vi "AutoBike FPGA.vi"() -> ()   [LabVIEW 2016]
doc: "The roboRIO FPGA Shipping Personality. This personality supports:\n- 8 Analog Input channels with 1 sample\n- 2 Analog Output channels with 1 sample\n- 30 Digital I/O channels with 1 sample\n- 1 RSL channel\n- 4 Relay channels\n- 1 Button\n- 3 LEDs\n- 1 Accelerometer\n- 13 PWM channels\n- 6 Encoder channels\n- 2 SPI channels\n- 2 I2C channels\n- 2 UART channels\n- 1 CAN channel\n- 2 Analog Input Interrupt\n- 5 Digital Input Interrupt\n- 1 Timer Interrupt"
uses:
  Sub VIs for FPGA/SubVIs needed for the customize FPGA VI/Utilities/Start Boolean.ctl
  <vilib>/Platform/TimedLoop/XDataNode/timing_clust.ctl
  <vilib>/Platform/TimedLoop/XDataNode/nitl_modes.ctl
  <vilib>/Platform/TimedLoop/XDataNode/wakeup.ctl
  <vilib>/rvi/Analysis/control/PID/Typedef/niFpgaPID_PIGains.ctl
  <vilib>/rvi/Analysis/control/PID/Typedef/niFpgaPID_OutputRange.ctl
  <vilib>/rvi/Emulation/niFpgaGetClockAttributes.vi
  <vilib>/rvi/Emulation/niFpgaSctlEmulationGetInTimedLoop.vi
  <vilib>/rvi/Emulation/niFpgaEmulationReportErrorSimple.vi
  <vilib>/rvi/eio/common/nirviEmuTemplateMethod_errors.vi
  <vilib>/rvi/Emulation/niFpgaCriticalErrorInLSC.vi
  <vilib>/rvi/Emulation/niFpgaProcessEmulError.vi
  <vilib>/rvi/Emulation/niFpgaEmulationIsFPGAContextNoSignature.vi
  <vilib>/rvi/errors/niFpgaSetErrorForExecOnDevCompSimple.vi
  <vilib>/rvi/eio/common/nirviEmuReportErrorAndStop.vi
  <vilib>/rvi/DataTransferAndStorage/Container/Common/niFpgaContainerGetUniqueNameForEmu.vi
  <vilib>/rvi/FIFO/Fifo_Resource/nirvififoEmulationSetSize.vi
  <vilib>/rvi/FIFO/Fifo_Resource/nirviFifoEmulationQueueMgr.vi
  <instcachedir>/0/nirviFifoEmulationQueueMgr_E5CAEC123FF24DC58D834DCA3CDAA9B5.lvgen/nirviFifoEmulationQueueMgr_E5CAEC123FF24DC58D834DCA3CDAA9B5_002.vi
  <vilib>/Utility/error.llb/Clear Errors.vi
  <vilib>/rvi/FIFO/Fifo_Resource/nirvififoEmulationCreateLock.vi
  <vilib>/rvi/FIFO/Fifo_Resource/nirvififoEmulationObtainLock.vi
  <vilib>/rvi/FIFO/Fifo_Resource/nirvififoEmulationReleaseLock.vi
  <vilib>/rvi/occurrence/nirviWaitOnOccurrenceBase.vi
  <vilib>/rvi/errors/nirviReportUnexpectedCaseInternalError.vi
  <vilib>/rvi/errors/nirviReportUnexpectedCaseInternalError (U32).vi
  <vilib>/rvi/FIFO/Fifo_Resource/nirvififoEmulationDetermineInputValidOut.vi
  <vilib>/rvi/Analysis/control/PID/SubVIs/niFpgaPID_PIWrapper.vi
  <vilib>/rvi/DataTransferAndStorage/Container/Common/niFpgaContainerSetEmuInfo.vi
  <vilib>/eio/EIONode/EIONode.xnode
  <vilib>/rvi/DataTransferAndStorage/Container/XNode/niFpgaContainer.xnode
  <vilib>/rvi/FIFO/Fifo_Resource/nirvififoEmulationRead.vi
  <vilib>/rvi/FIFO/Fifo_Resource/nirvififoEmulationWrite.vi
  <vilib>/Platform/TimedLoop/XDataNode/XDataNode.xnode
  <vilib>/rvi/LocalResourceManager/LocalResourceManager.xnode
  <vilib>/Platform/TimedLoop/XDataNode/XDNodeRunTimeDep.lvlib
panel:
  out "error":sgl
  in  "Control Loop Duty Cycle":sgl
  in  "Control Loop Direction":bool
  in  "Front Panel Duty Cycle":sgl
  in  "Front Panel Direction":bool
  in  "Shut Down BW":bool
  out "Duty cycle (steering)":sgl
  out "Steering angle(deg)":sgl
  in  "Duty Cycle in":sgl
  out "Current speed":sgl
  out "Duty cycle (BW)":sgl
  in  "Reference speed in km/h":sgl=15.0
  out "Filtered data":i32
  out "Value Channel 0":i32
  out "Channel 4 position":i32
  out "Channel 5 position":i32
  out "Channel 6 position":i32
  out "Channel 7 position":i32
  out "Position":i64
  in  "Stop encoder":bool
  in  "Reset counter":bool
  in  "Stop direction switch":bool
  in  "Switch direction":bool
  out "HallSensorValue":u8
  in  "Stop Hallsensor":bool
  out "dt":u32
  out "DIO.SPI_CS3:0.IN":u8 format="%08b"
  in  "DIO.SPI_CS3:0.DIR":u8 format="%08b"
  in  "DIO.SPI_CS3:0.OUT":u8 format="%08b"
  in  "IRQ.TIMER.SETTIME":T1
  in  "IRQ.TIMER.WRITE":u32
  out "IRQ.TIMER.READ":u32
  in  "IRQ.DI_BTN.NO":u8
  in  "IRQ.DI_BTN.CNT":u32
  in  "IRQ.DI_BTN.FALL":bool
  in  "IRQ.DI_BTN.RISE":bool
  in  "IRQ.DI_BTN.ENA":bool
  in  "IRQ.AI_B_0.HYSTERESIS":u16=17
  in  "IRQ.AI_B_1.HYSTERESIS":u16=17
  in  "IRQ.AI_B_1.NO":u8
  in  "IRQ.AI_B_0.NO":u8
  in  "IRQ.AI_B_1.THRESHOLD":u16
  in  "IRQ.AI_B_0.THRESHOLD":u16
  in  "IRQ.AI_B_3:0.CNFG":u8 format="%.0b"
  in  "IRQ.DIO_B_0.NO":u8
  in  "IRQ.DIO_B_1.NO":u8
  in  "IRQ.DIO_B_2.NO":u8
  in  "IRQ.DIO_B_3.NO":u8
  in  "IRQ.DIO_B_3.CNT":u32
  in  "IRQ.DIO_B_2.CNT":u32
  in  "IRQ.DIO_B_1.CNT":u32
  in  "IRQ.DIO_B_0.CNT":u32
  in  "IRQ.DIO_B_7:0.FALL":u8 format="%08b"
  in  "IRQ.DIO_B_7:0.RISE":u8 format="%08b"
  in  "IRQ.DIO_B_7:0.ENA":u8 format="%08b"
  in  "SPI.SPI.IRQ.NO":u8=15
  in  "SPI.B.IRQ.NO":u8=15
  out "DIO.DIO_9:8.IN":u8 format="%08b"
  in  "ENC.DIO_3.CNFG":u8 format="%08b"
  out "ENC.DIO_3.CNTR":u32
  out "ENC.DIO_3.STAT":u8 format="%08b"
  in  "ENC.DIO_4.CNFG":u8 format="%08b"
  out "ENC.DIO_4.CNTR":u32
  out "ENC.DIO_4.STAT":u8 format="%08b"
  in  "DIO.DIO_9:8.OUT":u8 format="%08b"
  in  "DIO.DIO_9:8.DIR":u8 format="%08b"
  in  "ENC.DIO_2.CNFG":u8 format="%08b"
  out "ENC.DIO_2.CNTR":u32
  out "ENC.DIO_2.STAT":u8 format="%08b"
  out "ENC.DIO_1.STAT":u8 format="%08b"
  out "ENC.DIO_1.CNTR":u32
  in  "ENC.DIO_1.CNFG":u8 format="%08b"
  out "DIO.DIO_7:0.IN":u8 format="%08b"
  in  "SYS.SELECTDIO":u8 format="%08b"
  in  "DIO.DIO_7:0.DIR":u8 format="%08b"
  in  "DIO.DIO_7:0.OUT":u8 format="%08b"
  out "ENC.DIO_0.STAT":u8 format="%08b"
  out "ENC.DIO_0.CNTR":u32
  in  "ENC.DIO_0.CNFG":u8 format="%08b"
  out "DI.BTN":u8 format="%08b"
  in  "DO.LED 5:0":u8 format="%06b"
  in  "DO.RSL.OUT":bool
  out "SPI.SPI.STAT":u8 format="%08b"
  in  "SPI.SPI.GO":T1
  in  "SPI.SPI.CNT":u16
  in  "SPI.SPI.CNFG":u16 format="%016b"
  out "SPI.SPI.DATI":u16
  in  "SPI.SPI.DATO":u16
  out "I2C.I2C.DATI":u8
  out "I2C.I2C.STAT":u8 format="%08b"
  in  "I2C.I2C.DATO":u8
  in  "I2C.I2CADDR":u8 format="%08b"
  in  "I2C.I2C.CNTR":u8
  in  "I2C.I2C.CNTL":u8 format="%08b"
  in  "I2C.I2C.CNFG":u8 format="%08b"
  in  "I2C.I2C.GO":T1
  out "ACC.Z.VAL":u16
  out "ACC.Y.VAL":u16
  out "ACC.X.VAL":u16
  in  "DO.RELAY.OUT":u8 format="%08b"
  out "SYS.ACC.RDY":bool
  out "SYS.RDY":bool
  in  "PWM.PWM_5.MAX":u16
  in  "PWM.PWM_5.CMP":u16
  in  "PWM.PWM_5.CNFG":u8 format="%08b"
  in  "PWM.PWM_5.CS":u8
  out "PWM.PWM_5.CNTR":u16
  in  "PWM.PWM_6.MAX":u16
  in  "PWM.PWM_6.CMP":u16
  in  "PWM.PWM_6.CNFG":u8 format="%08b"
  in  "PWM.PWM_6.CS":u8
  out "PWM.PWM_6.CNTR":u16
  in  "PWM.PWM_7.MAX":u16
  in  "PWM.PWM_7.CMP":u16
  in  "PWM.PWM_7.CNFG":u8 format="%08b"
  in  "PWM.PWM_7.CS":u8
  out "PWM.PWM_7.CNTR":u16
  in  "PWM.PWM_8.MAX":u16
  in  "PWM.PWM_8.CMP":u16
  in  "PWM.PWM_8.CNFG":u8 format="%08b"
  in  "PWM.PWM_8.CS":u8
  out "PWM.PWM_8.CNTR":u16
  in  "PWM.PWM_9.MAX":u16
  in  "PWM.PWM_9.CMP":u16
  in  "PWM.PWM_9.CNFG":u8 format="%08b"
  in  "PWM.PWM_9.CS":u8
  out "PWM.PWM_9.CNTR":u16
  in  "PWM.PWM_4.MAX":u16
  in  "PWM.PWM_4.CMP":u16
  in  "PWM.PWM_4.CNFG":u8 format="%08b"
  in  "PWM.PWM_4.CS":u8
  out "PWM.PWM_4.CNTR":u16
  in  "PWM.PWM_3.MAX":u16
  in  "PWM.PWM_3.CMP":u16
  in  "PWM.PWM_3.CNFG":u8 format="%08b"
  in  "PWM.PWM_3.CS":u8
  out "PWM.PWM_3.CNTR":u16
  in  "PWM.PWM_2.MAX":u16
  in  "PWM.PWM_2.CMP":u16
  in  "PWM.PWM_2.CNFG":u8 format="%08b"
  in  "PWM.PWM_2.CS":u8
  out "PWM.PWM_2.CNTR":u16
  in  "PWM.PWM_1.MAX":u16
  in  "PWM.PWM_1.CMP":u16
  in  "PWM.PWM_1.CNFG":u8 format="%08b"
  in  "PWM.PWM_1.CS":u8
  out "PWM.PWM_1.CNTR":u16
  out "PWM.PWM_0.CNTR":u16
  in  "PWM.PWM_0.CS":u8
  in  "PWM.PWM_0.CNFG":u8 format="%08b"
  in  "PWM.PWM_0.CMP":u16
  in  "PWM.PWM_0.MAX":u16
  in  "AO.B_0.VAL":u16
  in  "AO.B_1.VAL":u16
  in  "AO.SYS.GO":T1
  out "AO.SYS.STAT":bool
  out "AI.B_0.VAL":u16
  out "AI.B_1.VAL":u16
  out "AI.B_2.VAL":u16
  out "AI.B_3.VAL":u16
  out "AI.AI_0.VAL":u16
  out "AI.AI_1.VAL":u16
  out "AI.AI_2.VAL":u16
  out "AI.AI_3.VAL":u16
  out "SYS.AI.RDY":bool
  in  "SYS.SELECTB":u8 format="%08b"
  in  "DIO.B_7:0.OUT":u8 format="%08b"
  in  "DIO.B_7:0.DIR":u8 format="%08b"
  out "DIO.B_7:0.IN":u8 format="%08b"
  in  "DIO.B_15:8.OUT":u8 format="%08b"
  in  "DIO.B_15:8.DIR":u8 format="%08b"
  out "DIO.B_15:8.IN":u8 format="%08b"
  in  "SPI.B.DATO":u16
  out "SPI.B.DATI":u16
  in  "SPI.B.CNFG":u16 format="%016b"
  in  "SPI.B.CNT":u16
  in  "SPI.B.GO":T1
  out "SPI.B.STAT":u8 format="%08b"
  in  "PWM.B_0.MAX":u16
  in  "PWM.B_0.CMP":u16
  in  "PWM.B_0.CNFG":u8 format="%08b"
  in  "PWM.B_0.CS":u8
  out "PWM.B_0.CNTR":u16
  in  "PWM.B_1.CMP":u16
  in  "PWM.B_1.MAX":u16
  out "PWM.B_1.CNTR":u16
  in  "PWM.B_1.CNFG":u8 format="%08b"
  in  "PWM.B_1.CS":u8
  in  "PWM.B_2.CMP":u16
  in  "PWM.B_2.MAX":u16
  out "PWM.B_2.CNTR":u16
  in  "PWM.B_2.CNFG":u8 format="%08b"
  in  "PWM.B_2.CS":u8
  in  "I2C.B.DATO":u8
  out "I2C.B.DATI":u8
  in  "I2C.B.ADDR":u8 format="%08b"
  in  "I2C.B.CNTR":u8
  in  "I2C.B.CNTL":u8 format="%08b"
  out "I2C.B.STAT":u8 format="%08b"
  in  "I2C.B.CNFG":u8 format="%08b"
  in  "I2C.B.GO":T1
  in  "ENC.B.CNFG":u8 format="%08b"
  out "ENC.B.CNTR":u32
  out "ENC.B.STAT":u8 format="%08b"
  # "System"
  # "Onboard Devices"
  # "Connector B"
  # "DIO"
  # "SPI"
  # "PWM"
  # "I2C"
  # "AI"
  # "RELAY"
  # "RSL"
  # "Accelerometer"
  # "SPI Master"
  # "Analog Input"
  # "Analog Output"
  # "Digital I/O"
  # "Counters / PWM"
  # "Digital I/O"
  # "Encoders"
  # "IO Configuration"
  # "Buttons & LEDs"
  # "SPI CS DIO"
  # "Analog Interrupt"
  # "Digital Interrupt"
  # "Encoders"
  # "IO Configuration"
  # "Button Interrupt"
  # "I2C Master"
  # "FPGA Timer"
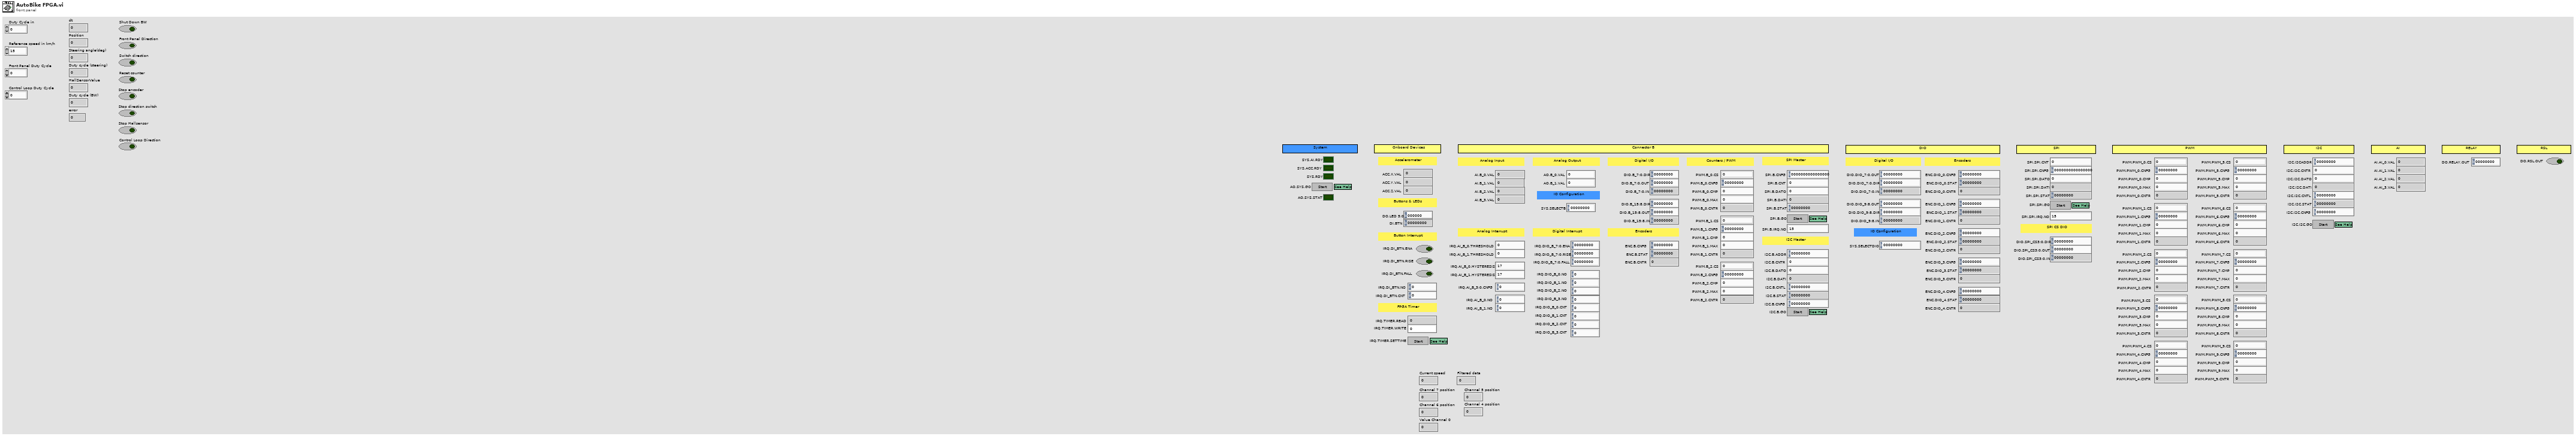
[diagram p1: front panel]
types:
  T1 = typedef "Start Boolean.ctl" = bool
  T2 = typedef "XDNodeRunTimeDep.lvlib/timing_clust.ctl" = cluster{"Expected End [f-1]":u64, "Actual End [f-1]":u64, "Finished Late? [f-1]":bool, "Expected End [i-1]":u64, "Actual End [i-1]":u64, "Finished Late? [i-1]":bool, "Expected Start [i]":u64, "Actual Start [i]":u64, "Expected Start [f]":u64, "Actual Start [f]":u64, "Source Name":string, "Structure Name":string, "Period":i64, "Deadline":i64, "Offset":i64, "Start":i64, "Priority":i32, "Timeout":i32, "Mode":T3, "Wakeup Reason":T4, "Error":errorcluster, "Source Type":string, "Secondary Source Type":string, "Global End Time":u64, "Global Start Time":u64, "Frame Duration":u64, "Iteration Duration":u64, "Assigned CPU":i32, "I/O Scan Engine Mode":u32}
  T3 = typedef "XDNodeRunTimeDep.lvlib/nitl_modes.ctl" = enum32{"No Change", "Process missed periods, maintain original phase", "Discard missed periods, maintain original phase", "Process missed periods, ignore original phase", "Discard missed periods, ignore original phase"}
  T4 = typedef "XDNodeRunTimeDep.lvlib/wakeup.ctl" = enum32{"Normal", "Aborted", "Asynchronous wakeup", "Timing source error", "Timed loop error", "Timeout"}
  T5 = typedef "niFpgaPID_OutputRange.ctl" = cluster{"output high (Inf)":sgl, "output low (-Inf)":sgl}
  T6 = typedef "niFpgaPID_PIGains.ctl" = cluster{"proportional gain":sgl, "integral gain":sgl}
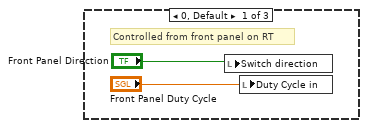
[diagram p2: hidden frame]
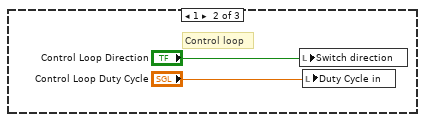
[diagram p3: hidden frame]
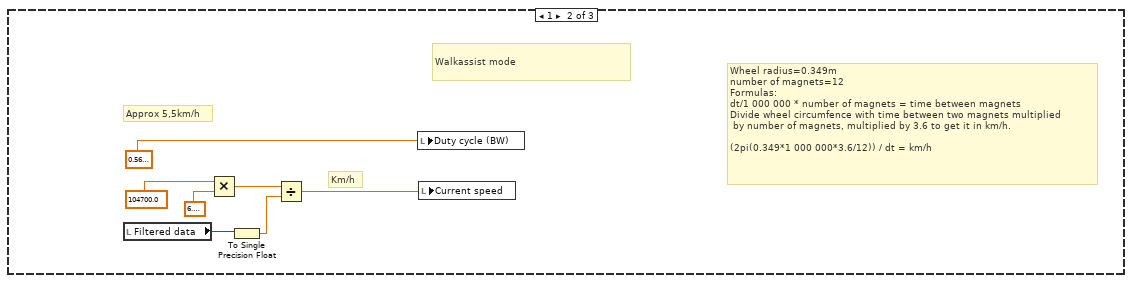
[diagram p4: hidden frame]
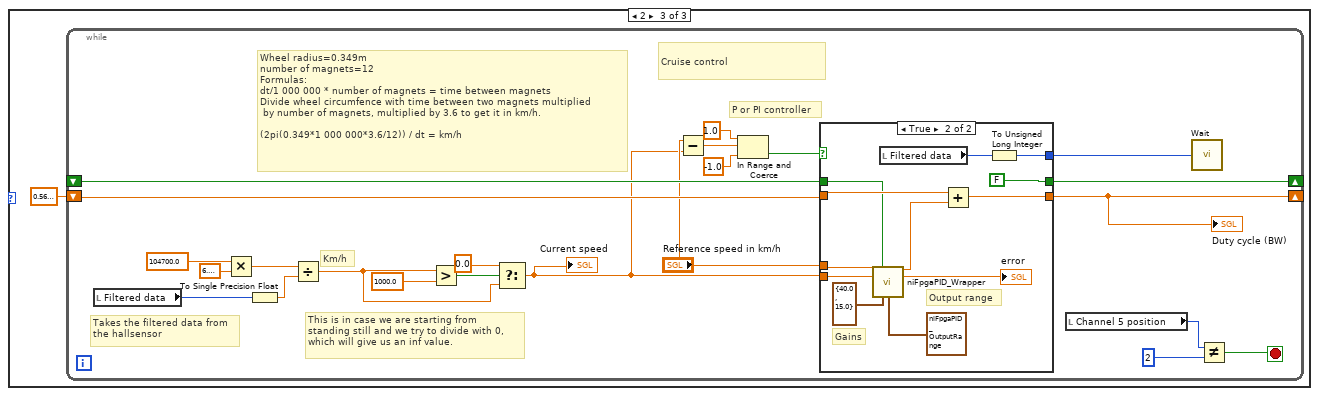
[diagram p5: hidden frame]
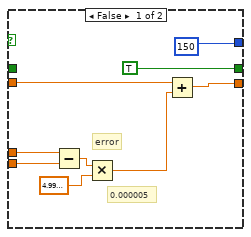
[diagram p6: hidden frame]
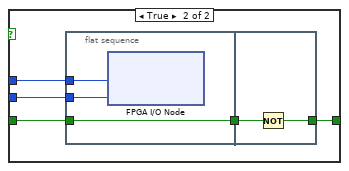
[diagram p13: hidden frame]
diagram:
  # "DONT USE PWN 1, IT IS CONNECTED ON THREE OUTS"
  # "The accelerometer nodes take some time before the FPGA can first read the values. This is because it takes time to read from the accelerometer. An iteration of the While Loop will not complete until the accelerometer values have been read.\n\nAfter the completion of the first iteration of the While Loop, all indicators have valid values."
  # "The analog output nodes take some time before the FPGA write the values to the pins. The GO and STAT registers are used to handshake between the FPGA and host. When the host wants the values to be written, the host sets the GO register to TRUE. If the host reads the STAT register before setting the value of the GO register, it can wait for the value of the STAT register to invert. The value inversion tells the host that the output values have been written."
  # "The FPGA timer fires the interrupt request (IRQ) when TIMER.Read counts down to zero. If TIMER.Read is not zero, it counts down to one per microsecond."
  # "The analog input nodes take some time before the FPGA can first read the values. This is because it takes time to set up the Analog-to-Digital converter (ADC) and convert the first reading. An iteration of the While Loop will not complete until all the analog input channels have been sampled.\n\nAfter the completion of the first iteration of the While Loop, all indicators have valid values."
  # "Note: On some hardware a \"ghosting effect\" may occur on any unconnected AI channels. For example, if channel AI0 is connected and channels AI1~AI7 are not connected the the value read at AI0 may be seen on indicators AI1~AI7. This is common for hardware that use a multiplexed (MUXed) Analog-to-Digital converter (ADC), because the input analog signal is used to charge a capacitor which does not discharge before the unconnected channel is read.\n\nYou can hide the \"ghosting effect\" by using an mask register. This register is used to decide when the indicator should be updated."
  # "The only interface that sends interrupts to the RT side. Timer interrupts, analog input interrupts, digital input interrupts, and SPI interrupt share this interface.\n\nAll interrupts work in sequence. One interrupt waits until the previous interrupt request (IRQ) gets acknowledged on the RT side."
  # "NOTE: The SYS.RDY boolean MUST exist and must become TRUE at some point otherwise the myRIO API will not function correctly."
  # "There is some delay between when the FPGA code starts and the analog inputs, accelerometer, and scaling values outputs are valid. If the host wants to ensure that there are valid values in theses registers it should wait for each subsystem to finish its initialization process. \n\nWhen all subsystems have finished initializinig, the SYS.RDY indicator will be true, which can be polled by the host to determine the status of the FPGA. Alternatively, the host can poll the individual SYS.xx.RDY indicators to determine the status of the individual subsystems.\n\nThis loop continues indefinitely, essentially making SYS.RDY a read-only register."
  n1 = flat-sequence {
    tunnel: [i64 0] -> w2
    tunnel: [TRUE ("DIO/DIO3")] -> w1
    tunnel: w2 -> [w29]
    tunnel: w1 -> [w28]
    frame #0 {
      # "Initialise"
    }
    frame #1 {
      n2 = while {
        shift-right: [w49] -> _
        shift-left: w28 -> [w51]
        stop <- "Stop Hallsensor" stop-if-true
        n3 = flat-sequence {
          tunnel: w51 -> [w54]
          tunnel: [w54] -> w48
          tunnel: [u8 0] -> w47
          tunnel: [w52] -> w46
          tunnel: w48 -> [w59]
          tunnel: w47 -> [w57]
          tunnel: w46 -> [w56]
          tunnel: [w58] -> w45
          tunnel: [w55] -> w44
          tunnel: [w81] -> w49
          tunnel: w45 -> [w81]
          tunnel: [w80] -> w43
          tunnel: w44 -> [w78]
          frame #0 {
            n4 = call "Tick Count4"() -> ("Tick Count(uSec)"=w52:u32)
          }
          frame #1 {
            n5 = node-c288() -> (w61:T2)  [unwired: 1 in]
            n6 = timed-loop {
              shift-right: [w65] -> _
              shift-left: w57 -> [w62]
              shift-right: [w70] -> w58
              shift-left: w59 -> [w73]
              timing: w61 -> [_]
              timing-out: [_] -> w60
              tunnel: w56 -> [w72]
              tunnel: [w72] -> w55
              stop <- w64 stop-if-true
              # "Calculates the time it takes to collect 2 rises, i.e one magnet"
              # "Reads the output from the hallsensor and outputs the number of change in rises"
              # "Hallsensor counter"
              n7 = xnode "FPGA I/O Node"() -> ("DIO/DIO8"=w70:bool)  [unwired: 1 in, 1 out]
              n8 = Exclusive Or(1:w73, 2:w70) -> (0:w68:bool)
              n9 = Not And(1:TRUE ("y"), 2:w70) -> (0:w69:bool)
              n10 = And(x=w69, y=w68) -> (x .and. y?=w67:bool)
              n11 = Increment(x=w62) -> (x+1=w66:u8)
              n12 = Select(t=w66, s=w67, f=w62) -> (s? t:f=w65:u8)
              "HallSensorValue" <- w65
              n13 = Equal?(x=u8 2, y=w65) -> (x = y?=w64:bool)
            }
            n14 = node-c288(w60) -> ()
          }
          frame #2 {
            n15 = call "Tick Count"() -> ("Tick Count(uSec)"=w79:u32)
            n16 = Subtract(x=w79, y=w78) -> (x-y=w80:u32)
          }
        }
        n17 = To Long Integer(number=w43) -> (32bit integer=w42:i32)
        n18 = call "Median filter.vi"("Rawdata"=w42) -> ("Filtered element"=w39:i32)  [unwired: 10 in]
        n19 = Equal To 0?(x=w39) -> (x = 0?=w41:bool)
        n20 = Select(t=1, s=w41, f=w39) -> (s? t:f=→"Filtered data":i32)
      }
      n21 = node-c288() -> (w31:T2)  [unwired: 1 in]
      n22 = node-c288() -> (w27:T2)  [unwired: 1 in]
      n23 = timed-loop {
        shift-right: [w92] -> _
        shift-left: w29 -> [w83]
        shift-right: [w89] -> _
        shift-left: _ -> [w87]
        shift-right: [w88] -> _
        shift-left: _ -> [w86]
        timing: w31 -> [_]
        timing-out: [_] -> w30
        stop <- "Stop encoder" stop-if-true
        # "Decoder, reads both signals and check if there is any change to any of the channels, if there is a change current A channel\nis compared to previous B channel to determine which direction the motor is going and updates the position counter\naccordingly. The counter is resetted each time the Main VI is deployed."
        # "Motor Decoder"
        n24 = xnode "FPGA I/O Node"() -> ("DIO/DIO0"=w89:bool, "DIO/DIO1"=w88:bool)  [unwired: 2 in, 2 out]
        n25 = Exclusive Or(1:w86, 2:w89) -> (0:w85:bool)
        n26 = Select(t=i64 0, s="Reset counter", f=w83) -> (s? t:f=w91:i64)
        n27 = Exclusive Or(1:w87, 2:w89) -> (0:w99:bool)
        n28 = Exclusive Or(1:w86, 2:w88) -> (0:w98:bool)
        n29 = Or(x=w99, y=w98) -> (x .or. y?=w84:bool)
        n30 = Select(t=i64 1, s=w85, f=i64 -1) -> (s? t:f=w94:i64)
        n31 = Add(x=w94, y=w91) -> (x+y=w93:i64)
        n32 = Select(t=w93, s=w84, f=w91) -> (s? t:f=w92:i64)
        "Position" <- w92
      }
      n33 = timed-loop {
        timing: w27 -> [_]
        timing-out: [_] -> w26
        stop <- "Stop direction switch" stop-if-true
        # "Switch the direction of the steering\nmotor."
        # "Switch direction"
        n34 = xnode "FPGA I/O Node"("DIO/DIO2"="Switch direction") -> ()  [unwired: 1 in, 1 out]
      }
      n35 = node-c288(w26) -> ()
      n36 = node-c288(w30) -> ()
    }
  }
  n37 = while {
    stop <- FALSE stop-if-true
    # "PWM signal to steering motor"
    n38 = flat-sequence {
      tunnel: [w107] -> w104
      tunnel: [w112] -> w106
      tunnel: w104 -> [w109]
      tunnel: w106 -> [w114]
      frame #0 {
        w107 = u32 40000 ("Freq")
        # "40000 ticks=1kHz"
        n39 = call "Loop Timer3"("Count(Ticks)"=w107) -> ()  [unwired: 1 out]
      }
      frame #1 {
        # "Too make sure 0 duty \ncycle is generated"
        n40 = local read "Duty cycle (steering)"() -> (w110:sgl)
        n41 = To Single Precision Float(number=w109) -> (single precision float=w108:sgl)
        n42 = Not Equal To 0?(x=w110) -> (x != 0?=w111:bool)
        n43 = Multiply(x=w110, y=w108) -> (x*y=w113:sgl)
        n44 = xnode "FPGA I/O Node"("PWM/PWM0"=w111) -> ()  [unwired: 1 in, 1 out]
        n45 = To Unsigned Long Integer(number=w113) -> (unsigned 32bit integer=w112:u32)
      }
      frame #2 {
        n46 = call "Wait3"("Count(Ticks)"=w114) -> ()  [unwired: 1 out]
      }
      frame #3 {
        n47 = xnode "FPGA I/O Node"("PWM/PWM0"=FALSE ("PWM/PWM8")) -> ()  [unwired: 1 in, 1 out]
      }
    }
  }
  n48 = while {
    stop <- FALSE stop-if-true
    # "PWM signal to backwheel motor"
    n49 = flat-sequence {
      tunnel: [w121] -> w117
      tunnel: w117 -> [w124]
      frame #0 {
        # "80 000ticks=500Hz"
        n50 = call "Loop Timer2"("Count(Ticks)"=u32 80000) -> ()  [unwired: 1 out]
      }
      frame #1 {
        n51 = local read "Duty cycle (BW)"() -> (w119:sgl)
        n52 = xnode "FPGA I/O Node"("PWM/PWM8"=TRUE) -> ()  [unwired: 1 in, 1 out]
        n53 = Multiply(x=w119, y=sgl 80000.0) -> (x*y=w122:sgl)
        n54 = To Unsigned Long Integer(number=w122) -> (unsigned 32bit integer=w121:u32)
      }
      frame #2 {
        n55 = call "Wait2"("Count(Ticks)"=w124) -> ()  [unwired: 1 out]
      }
      frame #3 {
        n56 = xnode "FPGA I/O Node"("PWM/PWM8"=FALSE) -> ()  [unwired: 1 in, 1 out]
      }
    }
  }
  n57 = while {
    stop <- FALSE stop-if-true
    # "Backwheel motor control"
    n58 = local read "Channel 5 position"() -> (w126:i32)
    n59 = case shown="0, Default" w126 {
      frame 0, Default {
        # "Wheel radius=0.349m\nnumber of magnets=12\nFormulas:\ndt/1 000 000 * number of magnets = time between magnets\nDivide wheel circumfence with time between two magnets multiplied\n by number of magnets, multiplied by 3.6 to get it in km/h.\n\n(2pi(0.349*1 000 000*3.6/12)) / dt = km/h"
        # "Takes the filtered data from\nthe hallsensor"
        # "Km/h"
        # "Standing still"
        n60 = local read "Filtered data"() -> (w129:i32)
        n61 = Multiply(x=sgl 104700.0, y=sgl 6.2831855) -> (x*y=w135:sgl)
        n62 = To Single Precision Float(number=w129) -> (single precision float=w130:sgl)
        n63 = Divide(x=w135, y=w130) -> (x/y=w131:sgl)
        n64 = Greater?(x=w131, y=sgl 1000.0) -> (0:w133:bool)
        n65 = local write "Duty cycle (BW)"(sgl 0.5 ("Duty cycle out 2")) -> ()
        n66 = Select(t=sgl 0.0, s=w133, f=w131) -> (s? t:f=w128:sgl)
        n67 = local write "Current speed"(w128) -> ()
      }
      frame 1 {
        # "Wheel radius=0.349m\nnumber of magnets=12\nFormulas:\ndt/1 000 000 * number of magnets = time between magnets\nDivide wheel circumfence with time between two magnets multiplied\n by number of magnets, multiplied by 3.6 to get it in km/h.\n\n(2pi(0.349*1 000 000*3.6/12)) / dt = km/h"
        # "Walkassist mode"
        # "Approx 5,5km/h"
        # "Km/h"
        n68 = local read "Filtered data"() -> (w142:i32)
        n69 = Multiply(x=sgl 104700.0, y=sgl 6.2831855) -> (x*y=w143:sgl)
        n70 = To Single Precision Float(number=w142) -> (single precision float=w141:sgl)
        n71 = Divide(x=w143, y=w141) -> (x/y=w140:sgl)
        n72 = local write "Duty cycle (BW)"(sgl 0.56 ("Duty cycle out")) -> ()
        n73 = local write "Current speed"(w140) -> ()
      }
      frame 2 {
        n74 = while {
          shift-right: [w157] -> _
          shift-left: sgl 0.56 -> [w156]
          shift-right: [w155] -> _
          shift-left: _ -> [w154]
          stop <- w158 stop-if-true
          # "P or PI controller"
          # "This is in case we are starting from\nstanding still and we try to divide with 0, \nwhich will give us an inf value."
          # "Cruise control"
          # "Takes the filtered data from\nthe hallsensor"
          # "Wheel radius=0.349m\nnumber of magnets=12\nFormulas:\ndt/1 000 000 * number of magnets = time between magnets\nDivide wheel circumfence with time between two magnets multiplied\n by number of magnets, multiplied by 3.6 to get it in km/h.\n\n(2pi(0.349*1 000 000*3.6/12)) / dt = km/h"
          # "Km/h"
          n75 = local read "Filtered data"() -> (w161:i32)
          n76 = Multiply(x=sgl 104700.0, y=sgl 6.2831855) -> (x*y=w167:sgl)
          n77 = To Single Precision Float(number=w161) -> (single precision float=w162:sgl)
          n78 = Divide(x=w167, y=w162) -> (x/y=w163:sgl)
          n79 = Greater?(x=w163, y=sgl 1000.0) -> (0:w165:bool)
          n80 = Select(t=sgl 0.0, s=w165, f=w163) -> (s? t:f=w152:sgl)
          "Current speed" <- w152
          n81 = Subtract(x="Reference speed in km/h", y=w152) -> (x-y=w151:sgl)
          n82 = In Range and Coerce(upper limit=sgl 1.0, x=w151, lower limit=sgl -1.0) -> (In Range?=w148:bool)  [unwired: 1 out]
          n83 = case shown="True" w148 {
            tunnel: [w178 w190] -> w157
            tunnel: "Reference speed in km/h" -> [w174 w188]
            tunnel: w156 -> [w176 w189]
            tunnel: w152 -> [w173 w187]
            tunnel: [TRUE FALSE] -> w155
            tunnel: w154 -> [_ w181]
            tunnel: [u32 150 ("Count(uSec)") w180] -> w147
            frame False {
              # "error"
              # "0.000005"
              n84 = Subtract(x=w174, y=w173) -> (x-y=w175:sgl)
              n85 = Multiply(x=w175, y=sgl 5e-07 ("P gain")) -> (x*y=w177:sgl)
              n86 = Add(x=w176, y=w177) -> (x+y=w178:sgl)
            }
            frame True {
              # "Gains"
              # "Output range"
              n87 = call-poly <vilib>:"niFpgaPID_Wrapper.vi"("setpoint"=w188, "reset? (F)"=w181, "process variable"=w187, "gains"=T6 {"proportional gain"=40.0, "integral gain"=15.0}, "output range"=T5 {"output high (Inf)"=0.0001, "output low (-Inf)"=-0.0001}) -> ("output"=w186:sgl, "error"=→"error":sgl)  [unwired: 8 in, 1 out]
              n88 = local read "Filtered data"() -> (w179:i32)
              n89 = Add(x=w189, y=w186) -> (x+y=w190:sgl)
              n90 = To Unsigned Long Integer(number=w179) -> (unsigned 32bit integer=w180:u32)
            }
          }
          "Duty cycle (BW)" <- w157
          n91 = local read "Channel 5 position"() -> (w160:i32)
          n92 = call "Wait"("Count(uSec)"=w147) -> ()  [unwired: 1 out]
          n93 = Not Equal?(x=w160, y=2) -> (x != y?=w158:bool)
        }
      }
    }
  }
  n94 = while {
    stop <- FALSE stop-if-true
    # "Host Synchronization"
    n95 = local read "SYS.ACC.RDY"() -> (w192:bool)
    n96 = local read "SYS.AI.RDY"() -> (w194:bool)
    n97 = Compound Arithmetic op=AND(w194, w192) -> (→"SYS.RDY":bool)
  }
  n98 = while {
    stop <- FALSE stop-if-true
    # "Interrupt to RT"
    n99 = xnode ("FIFO Method Node")("Timeout"=-1) -> ("Element"=w197:u8)  [unwired: 1 in, 2 out]
    n100 = call <vilib>:"niFPGA Interrupt.vi"("Wait Until Cleared (F)"=TRUE, "IRQ Number (0)"=w197) -> ()  [unwired: 1 in]
  }
  n101 = while {
    stop <- FALSE stop-if-true
    # "Receiver"
    n102 = call "Receiver.vi"() -> ("Channel 7 position"=→"Channel 7 position":i32, "Channel 6 position"=→"Channel 6 position":i32, "Channel 5 position"=w202:i32, "Channel 4 position"=→"Channel 4 position":i32, "Value Channel 0"=→"Value Channel 0":i32)  [unwired: 7 in]
    n103 = Select(t=0, s="Shut Down BW", f=w202) -> (s? t:f=→"Channel 5 position":i32)
  }
  n104 = while {
    stop <- FALSE stop-if-true
    # "Steering motor"
    n105 = local read "Switch direction"() -> (w213:bool)
    n106 = local read "Position"() -> (w210:i64)
    n107 = call "Steering motor.vi"("Steering position (in pulses)"=w210, "Duty Cycle in"="Duty Cycle in", "Switch direction"=w213) -> ("Duty Cycle out"=→"Duty cycle (steering)":sgl, "Steering angle(deg)"=→"Steering angle(deg)":sgl)  [unwired: 7 in]
  }
  n108 = while {
    stop <- FALSE stop-if-true
    # "RC steering motor switch"
    n109 = local read "Channel 6 position"() -> (w215:i32)
    n110 = case shown="2" w215 {
      frame 0, Default {
        # "Controlled from front panel on RT"
        n111 = local write "Switch direction"("Front Panel Direction") -> ()
        n112 = local write "Duty Cycle in"("Front Panel Duty Cycle") -> ()
      }
      frame 1 {
        # "Control loop"
        n113 = local write "Switch direction"("Control Loop Direction") -> ()
        n114 = local write "Duty Cycle in"("Control Loop Duty Cycle") -> ()
      }
      frame 2 {
        n115 = local read "Value Channel 0"() -> (w222:i32)
        n116 = call "RC steering motor interpolation.vi"("Value Channel 0"=w222) -> ("Numeric"=w221:sgl, "Boolean"=w220:bool)  [unwired: 9 in]
        n117 = local write "Duty Cycle in"(w221) -> ()
        n118 = local write "Switch direction"(w220) -> ()
      }
    }
  }
  n119 = while {
    stop <- FALSE stop-if-true
    # "Timer"
    n120 = local read "IRQ.TIMER.READ"() -> (w226:u32)
    n121 = Select(t="IRQ.TIMER.WRITE", s="IRQ.TIMER.SETTIME", f=w226) -> (s? t:f=w224:u32)
    n122 = case shown="Default" w224 {
      selector: w224 -> [w230 w233]
      tunnel: [w230 w231] -> w223
      frame 0 {
      }
      frame Default {
        n123 = Decrement(x=w233) -> (x-1=w232:u32)
        n124 = case shown="0" w232 {
          selector: w232 -> [w234 w237]
          tunnel: [w234 w237] -> w231
          frame Default {
          }
          frame 0 {
            w236 = u8 0  # Reserved for Timer IRQ
            n125 = xnode ("FIFO Method Node")("Element"=w236, "Timeout"=-1) -> ()  [unwired: 1 in, 2 out]
          }
        }
      }
    }
    "IRQ.TIMER.READ" <- w223
    n126 = call "Loop Timer"("Count(uSec)"=u8 1 ("Count(mSec)")) -> ()  [unwired: 1 out]
  }
  n127 = xnode "VI-Defined FIFO Configuration"() -> ("FIFO Out"=w4:refnum<k21>)
  n128 = while {
    tunnel: w4 -> [w246]
    i -> [w260]
    stop <- FALSE stop-if-true
    # "Analog Input"
    n129 = Greater Than 0?(x=w260) -> (x > 0?=→"SYS.AI.RDY":bool)
    n130 = xnode "FPGA I/O Node"() -> ("MXP/AI0"=w239:u16, "MXP/AI1"=w238:u16, "MXP/AI2"=→"AI.B_2.VAL":u16, "MXP/AI3"=→"AI.B_3.VAL":u16, "AnalogIn0"=→"AI.AI_0.VAL":u16, "AnalogIn1"=→"AI.AI_1.VAL":u16, "AnalogIn2"=→"AI.AI_2.VAL":u16, "AnalogIn3"=→"AI.AI_3.VAL":u16)  [unwired: 8 in, 8 out]
    "AI.B_0.VAL" <- w239
    "AI.B_1.VAL" <- w238
    n131 = Number To Boolean Array(number="IRQ.AI_B_3:0.CNFG") -> (Boolean array=w247:bool[])
    n132 = Index Array(array=w247) -> (element #1=w249:bool, element #2=w250:bool, element #3=w252:bool, element #4=w253:bool)  [unwired: 4 in]
    n133 = call "Check AI IRQ.vi"("Hysteresis"="IRQ.AI_B_1.HYSTERESIS", "FIFO In"=w246, "IRQ Number"="IRQ.AI_B_1.NO", "Threshold"="IRQ.AI_B_1.THRESHOLD", "Analog Value"=w238, "Rising Edge?"=w253, "Enable Interrupt?"=w252) -> ()  [unwired: 5 in]
    n134 = call "Check AI IRQ.vi"("Hysteresis"="IRQ.AI_B_0.HYSTERESIS", "FIFO In"=w246, "IRQ Number"="IRQ.AI_B_0.NO", "Threshold"="IRQ.AI_B_0.THRESHOLD", "Analog Value"=w239, "Rising Edge?"=w250, "Enable Interrupt?"=w249) -> ()  [unwired: 5 in]
  }
  n135 = while {
    stop <- FALSE stop-if-true
    # "Analog Output"
    n136 = feedback #1(FALSE) -> (w264:bool)
    n137 = case shown="False" "AO.SYS.GO" {
      tunnel: "AO.B_0.VAL" -> [_ w274]
      tunnel: "AO.B_1.VAL" -> [_ w273]
      tunnel: w264 -> [w269 w272]
      tunnel: [w269 w270] -> w262
      frame False {
      }
      frame True {
        n138 = flat-sequence {
          tunnel: w274 -> [w277]
          tunnel: w273 -> [w276]
          tunnel: w272 -> [w275]
          tunnel: [w275] -> w271
          tunnel: w271 -> [w279]
          tunnel: [w278] -> w270
          frame #0 {
            n139 = xnode "FPGA I/O Node"("MXP/AO0"=w277, "MXP/AO1"=w276) -> ()  [unwired: 2 in, 2 out]
          }
          frame #1 {
            n140 = Not(x=w279) -> (.not. x?=w278:bool)
          }
        }
      }
    }
    "AO.SYS.STAT" <- w262
    n141 = feedback-in #1(w262) -> ()
  }
  n142 = while {
    i -> [w287]
    stop <- FALSE stop-if-true
    # "Onboard Accelerometer"
    n143 = xnode "FPGA I/O Node"() -> ("AccelerationX"=w285:i16, "AccelerationY"=w284:i16, "AccelerationZ"=w283:i16)  [unwired: 3 in, 3 out]
    n144 = Greater Than 0?(x=w287) -> (x > 0?=→"SYS.ACC.RDY":bool)
    n145 = To Unsigned Word Integer(number=w285) -> (unsigned 16bit integer=→"ACC.X.VAL":u16)
    n146 = To Unsigned Word Integer(number=w284) -> (unsigned 16bit integer=→"ACC.Y.VAL":u16)
    n147 = To Unsigned Word Integer(number=w283) -> (unsigned 16bit integer=→"ACC.Z.VAL":u16)
  }
  n148 = xnode "VI-Defined FIFO Configuration"() -> ("FIFO Out"=w3:refnum<k21>)
  n149 = node-c288() -> (w9:T2)  [unwired: 1 in]
  n150 = timed-loop {
    timing: w9 -> [_]
    timing-out: [_] -> w8
    tunnel: w3 -> [w294]
    stop <- FALSE stop-if-true
    # "Button IRQ"
    # "Onboard DIO"
    n151 = xnode "FPGA I/O Node"() -> ("User Button"=w295:bool)  [unwired: 1 in, 1 out]
    n152 = Number To Boolean Array(number="DO.LED 5:0") -> (Boolean array=w305:bool[])
    n153 = Index Array(array=w305) -> (element #1=w303:bool, element #2=w302:bool, element #3=w301:bool, element #4=w300:bool, element #5=w299:bool, element #6=w298:bool)  [unwired: 6 in]
    n154 = Build Array(w295) -> (w297:bool[])
    n155 = call "DIO IRQ 1-bit.vi"("IRQ.NO"="IRQ.DI_BTN.NO", "IRQ.CNT"="IRQ.DI_BTN.CNT", "FIFO in"=w294, "IRQ.FALL"="IRQ.DI_BTN.FALL", "IRQ.RISE"="IRQ.DI_BTN.RISE", "IRQ.ENA"="IRQ.DI_BTN.ENA", "DIO"=w295) -> ()  [unwired: 5 in]
    n156 = Boolean Array To Number(Boolean array=w297) -> (number=→"DI.BTN":u8)
    n157 = xnode "FPGA I/O Node"("Radio LED Green"=w303, "Radio LED Red"=w302, "Comm LED Green"=w301, "Comm LED Red"=w300, "Mode LED Green"=w299, "Mode LED Red"=w298) -> ()  [unwired: 6 in, 6 out]
  }
  n158 = while {
    stop <- FALSE stop-if-true
    # "Button SCTL Interrupt Buffer"
    n159 = feedback #2(u8 0 ("Element")) -> (w311:u8)
    n160 = feedback #3(FALSE ("Timed Out?")) -> (w315:bool)
    n161 = case shown="False" w315 {
      tunnel: [w317 w319] -> w312
      tunnel: w311 -> [_ w319]
      frame False {
        n162 = xnode ("FIFO Read")("Timeout"=-1) -> ("Element"=w317:u8)  [unwired: 1 in, 2 out]
      }
      frame True {
      }
    }
    n163 = feedback-in #2(w312) -> ()
    n164 = xnode ("FIFO Method Node")("Element"=w312, "Timeout"=0) -> ("Timed Out?"=w313:bool)  [unwired: 1 in, 1 out]
    n165 = feedback-in #3(w313) -> ()
  }
  n166 = node-c288(w8) -> ()
  n167 = xnode "VI-Defined FIFO Configuration"() -> ("FIFO Out"=w7:refnum<k21>)
  n168 = xnode "VI-Defined FIFO Configuration"() -> ("FIFO Out"=w5:refnum<k21>)
  n169 = node-c288() -> (w23:T2)  [unwired: 1 in]
  n170 = timed-loop {
    timing: w23 -> [_]
    timing-out: [_] -> w22
    tunnel: w7 -> [w356]
    tunnel: w5 -> [w344]
    stop <- _ stop-if-true
    # "DIO/ IRQ"
    # "DIO / Encoder"
    # "DIO / I2C Master"
    # "DIO / PWM"
    # "DIO"
    # "DIO"
    # "DIO/ SPI Master"
    # "Connector MXP DIO"
    n171 = call "Split HDC Bank1 DIO.vi"("IN 7:0"="DIO.B_7:0.OUT") -> ("OUT 3:0"=w444:fxp<+,4,4>, "OUT 4"=w359:bool, "OUT 7:5"=w441:fxp<+,3,3>)
    n172 = call "Split HDC Bank1 DIO.vi"("IN 7:0"="DIO.B_7:0.DIR") -> ("OUT 3:0"=w443:fxp<+,4,4>, "OUT 4"=w442:bool, "OUT 7:5"=w440:fxp<+,3,3>)
    n173 = call "Split HDC Function Select.vi"("IN 7:0"="SYS.SELECTB") -> ("OUT 1:0"=w380:fxp<+,2,2>, "OUT 7"=w375:bool, "OUT 2"=w379:bool, "OUT 3"=w378:bool, "OUT 4"=w377:bool, "OUT 5"=w376:bool)
    n174 = call "DIO 4-bit.vi"("DIO0 Refnum"=refnum<k21> "MXP/DIO0", "DIO1 Refnum"=refnum<k21> "MXP/DIO1", "DIO2 Refnum"=refnum<k21> "MXP/DIO2", "DIR 3:0"=w443, "OUT 3:0"=w444, "DIO3 Refnum"=refnum<k21> "MXP/DIO3") -> ("IN 3:0"=w355:fxp<+,4,4>)  [unwired: 5 in]
    n175 = call "DIO 1-bit.vi"("DIR"=w442, "OUT"=w359, "DIO Refnum"=refnum<k21> "MXP/DIO4") -> ("IN"=w416:bool)  [unwired: 8 in]
    n176 = call "DIO_SPI.vi"("DIO.2:0.OUT"=w441, "DIO.2:0.DIR"=w440, "SPI.CNT"="SPI.B.CNT", "SPI.CNFG"="SPI.B.CNFG", "SPI.DATO"="SPI.B.DATO", "SPI.GO"="SPI.B.GO", "DIO.2/SPI.MOSI Refnum"=refnum<k21> "MXP/DIO7" ("DIO.2/SPI.SCLK"), "SELECT.1:0"=w380, "DIO.1/SPI.MISO Refnum"=refnum<k21> "MXP/DIO6" ("DIO.1/SPI.MOSI"), "DIO.0/SPI.SCLK Refnum"=refnum<k21> "MXP/DIO5" ("DIO.0/SPI.MISO")) -> ("DIO.2:0.IN"=w415:fxp<+,3,3>, "SPI.DATI"=→"SPI.B.DATI":u16, "SPI.STAT"=w358:u8)  [unwired: 7 in]
    "SPI.B.STAT" <- w358
    n177 = call "SPI IRQ.vi"("SPI.A.IRQ.NO"="SPI.B.IRQ.NO", "SPI.STAT"=w358, "FIFO In"=w356) -> ()  [unwired: 9 in]
    n178 = call "Join HDC Bank1 DIO.vi"("IN 7:5"=w415, "IN 4"=w416, "IN 3:0"=w355) -> ("OUT 7:0"=→"DIO.B_7:0.IN":u8)
    n179 = Number To Boolean Array(number="IRQ.DIO_B_7:0.ENA") -> (Boolean array=w341:bool[])
    n180 = Number To Boolean Array(number="IRQ.DIO_B_7:0.RISE") -> (Boolean array=w332:bool[])
    n181 = Number To Boolean Array(number="IRQ.DIO_B_7:0.FALL") -> (Boolean array=w327:bool[])
    n182 = Index Array(array=w341) -> (element #1=w342:bool, element #2=w340:bool, element #3=w339:bool, element #4=w338:bool)  [unwired: 4 in]
    n183 = Index Array(array=w332) -> (element #1=w331:bool, element #2=w333:bool, element #3=w334:bool, element #4=w335:bool)  [unwired: 4 in]
    n184 = Index Array(array=w327) -> (element #1=w328:bool, element #2=w326:bool, element #3=w325:bool, element #4=w324:bool)  [unwired: 4 in]
    n185 = Build Array(w342, w340, w339, w338) -> (w343:bool[])
    n186 = Build Array(w331, w333, w334, w335) -> (w330:bool[])
    n187 = Build Array(w328, w326, w325, w324) -> (w329:bool[])
    n188 = Build Array("IRQ.DIO_B_0.CNT", "IRQ.DIO_B_1.CNT", "IRQ.DIO_B_2.CNT", "IRQ.DIO_B_3.CNT") -> (w350:u32[])
    n189 = Build Array("IRQ.DIO_B_0.NO", "IRQ.DIO_B_1.NO", "IRQ.DIO_B_2.NO", "IRQ.DIO_B_3.NO") -> (w345:u8[])
    n190 = Boolean Array To Number(Boolean array=w343) -> (number=w336:fxp<+,4,4>)
    n191 = Boolean Array To Number(Boolean array=w330) -> (number=w321:fxp<+,4,4>)
    n192 = Boolean Array To Number(Boolean array=w329) -> (number=w320:fxp<+,4,4>)
    n193 = call "DIO IRQ 4-bit.vi"("IRQ NO"=w345, "IRQ CNT"=w350, "FIFO In"=w344, "IRQ.FALL"=w320, "IRQ.RISE"=w321, "IRQ.ENA"=w336, "IN 3:0"=w355) -> ()  [unwired: 5 in]
    n194 = call "Split HDC Bank2 DIO.vi"("IN 7:0"="DIO.B_15:8.OUT") -> ("OUT 5"=w361:bool, "OUT 7:6"=w385:fxp<+,2,2>, "OUT 4:3"=w363:fxp<+,2,2>, "OUT 2"=w365:bool, "OUT 0"=w369:bool, "OUT 1"=w368:bool)  [unwired: 2 in]
    n195 = call "Split HDC Bank2 DIO.vi"("IN 7:0"="DIO.B_15:8.DIR") -> ("OUT 5"=w360:bool, "OUT 7:6"=w384:fxp<+,2,2>, "OUT 4:3"=w362:fxp<+,2,2>, "OUT 2"=w364:bool, "OUT 0"=w367:bool, "OUT 1"=w366:bool)  [unwired: 2 in]
    n196 = call "DIO_PWM.vi"("DIO.OUT"=w369, "DIO.DIR"=w367, "PWM.CS"="PWM.B_0.CS", "PWM.CNFG"="PWM.B_0.CNFG", "PWM.CMP"="PWM.B_0.CMP", "PWM.MAX"="PWM.B_0.MAX", "DIO/PWM"=refnum<k21> "MXP/DIO8", "SELECT"=w379) -> ("DIO.IN"=w374:bool, "PWM.CNTR"=→"PWM.B_0.CNTR":u16)  [unwired: 10 in]
    n197 = call "DIO_PWM.vi"("DIO.OUT"=w368, "DIO.DIR"=w366, "PWM.CS"="PWM.B_1.CS", "PWM.CNFG"="PWM.B_1.CNFG", "PWM.CMP"="PWM.B_1.CMP", "PWM.MAX"="PWM.B_1.MAX", "DIO/PWM"=refnum<k21> "MXP/DIO9", "SELECT"=w378) -> ("DIO.IN"=w373:bool, "PWM.CNTR"=→"PWM.B_1.CNTR":u16)  [unwired: 10 in]
    n198 = call "DIO_PWM.vi"("DIO.OUT"=w365, "DIO.DIR"=w364, "PWM.CS"="PWM.B_2.CS", "PWM.CNFG"="PWM.B_2.CNFG", "PWM.CMP"="PWM.B_2.CMP", "PWM.MAX"="PWM.B_2.MAX", "DIO/PWM"=refnum<k21> "MXP/DIO10", "SELECT"=w377) -> ("DIO.IN"=w372:bool, "PWM.CNTR"=→"PWM.B_2.CNTR":u16)  [unwired: 10 in]
    n199 = call "DIO_Encoder.vi"("DIO.1:0.OUT"=w363, "DIO.1:0.DIR"=w362, "QE.CNFG"="ENC.B.CNFG", "DIO.1/QE.B"=refnum<k21> "MXP/DIO12", "SELECT"=w376, "DIO.0/QE.A"=refnum<k21> "MXP/DIO11") -> ("DIO.1:0.IN"=w371:fxp<+,2,2>, "QE.CNTR"=→"ENC.B.CNTR":u32, "QE.STAT"=→"ENC.B.STAT":u8)  [unwired: 11 in]
    n200 = call "DIO 1-bit.vi"("DIR"=w360, "OUT"=w361, "DIO Refnum"=refnum<k21> "MXP/DIO13") -> ("IN"=w370:bool)  [unwired: 8 in]
    n201 = call "DIO_I2C.vi"("DIO.1:0.OUT"=w385, "DIO.1:0.DIR"=w384, "I2C.CNFG"="I2C.B.CNFG", "I2C.CNTL"="I2C.B.CNTL", "I2C.ADDR"="I2C.B.ADDR", "I2C.DATO"="I2C.B.DATO", "DIO.1/I2C.SDA"=refnum<k21> "MXP/DIO15" ("DIO.1/I2C.SCL"), "I2C.CNTR"="I2C.B.CNTR", "DIO.0/I2C.SCL"=refnum<k21> "MXP/DIO14" ("DIO.0/I2C.SDA"), "Execute?"="I2C.B.GO", "SELECT"=w375) -> ("DIO.1:0.IN"=w382:fxp<+,2,2>, "I2C.DATI"=→"I2C.B.DATI":u8, "I2C.STAT"=→"I2C.B.STAT":u8)  [unwired: 6 in]
    n202 = call "Join HDC Bank2 DIO.vi"("IN 7:6"=w382, "IN 5"=w370, "IN 4:3"=w371, "IN 0"=w374, "IN 2"=w372, "IN 1"=w373) -> ("OUT 7:0"=→"DIO.B_15:8.IN":u8)  [unwired: 4 in]
  }
  n203 = while {
    stop <- FALSE stop-if-true
    # "Connector A SPI SCTL Interrupt Buffer"
    n204 = feedback #4(u8 0 ("Element")) -> (w449:u8)
    n205 = feedback #5(FALSE ("Timed Out?")) -> (w453:bool)
    n206 = case shown="False" w453 {
      tunnel: [w455 w457] -> w450
      tunnel: w449 -> [_ w457]
      frame False {
        n207 = xnode ("FIFO Method Node")("Timeout"=-1) -> ("Element"=w455:u8)  [unwired: 1 in, 2 out]
      }
      frame True {
      }
    }
    n208 = feedback-in #4(w450) -> ()
    n209 = xnode ("FIFO Method Node")("Element"=w450, "Timeout"=0) -> ("Timed Out?"=w451:bool)  [unwired: 1 in, 1 out]
    n210 = feedback-in #5(w451) -> ()
  }
  n211 = while {
    stop <- FALSE stop-if-true
    # "Connector A DIO SCTL Interrupt Buffer"
    n212 = feedback #6(u8 0 ("Element")) -> (w460:u8)
    n213 = feedback #7(FALSE ("Timed Out?")) -> (w464:bool)
    n214 = case shown="False" w464 {
      tunnel: [w466 w468] -> w461
      tunnel: w460 -> [_ w468]
      frame False {
        n215 = xnode ("FIFO Method Node")("Timeout"=-1) -> ("Element"=w466:u8)  [unwired: 1 in, 2 out]
      }
      frame True {
      }
    }
    n216 = feedback-in #6(w461) -> ()
    n217 = xnode ("FIFO Method Node")("Element"=w461, "Timeout"=0) -> ("Timed Out?"=w462:bool)  [unwired: 1 in, 1 out]
    n218 = feedback-in #7(w462) -> ()
  }
  n219 = node-c288(w22) -> ()
  n220 = node-c288() -> (w17:T2)  [unwired: 1 in]
  n221 = timed-loop {
    timing: w17 -> [_]
    timing-out: [_] -> w16
    stop <- FALSE stop-if-true
    # "Detta ska vara dio4"
    # "DIO"
    n222 = call "Split HDC Bank3 DIO.vi"("IN 7:0"="DIO.DIO_7:0.OUT") -> ("OUT 1:0"=w484:fxp<+,2,2>, "OUT 3:2"=w483:fxp<+,2,2>, "OUT 5:4"=w482:fxp<+,2,2>, "OUT 7:6"=w474:fxp<+,2,2>)
    n223 = call "Split HDC Bank3 DIO.vi"("IN 7:0"="DIO.DIO_7:0.DIR") -> ("OUT 1:0"=w480:fxp<+,2,2>, "OUT 3:2"=w479:fxp<+,2,2>, "OUT 5:4"=w478:fxp<+,2,2>, "OUT 7:6"=w473:fxp<+,2,2>)
    n224 = Number To Boolean Array(number="SYS.SELECTDIO") -> (Boolean array=w515:bool[])
    n225 = Index Array(array=w515) -> (element #1=w514:bool, element #2=w511:bool, element #3=w502:bool, element #4=w491:bool, element #5=w490:bool)  [unwired: 5 in]
    n226 = call "DIO_Encoder.vi"("DIO.1:0.OUT"=w474, "DIO.1:0.DIR"=w473, "QE.CNFG"="ENC.DIO_3.CNFG", "DIO.1/QE.B"=refnum<k21> "DIO/DIO7" ("DIO Refnum"), "SELECT"=w491, "DIO.0/QE.A"=refnum<k21> "DIO/DIO6" ("DIO Refnum")) -> ("DIO.1:0.IN"=w472:fxp<+,2,2>, "QE.CNTR"=→"ENC.DIO_3.CNTR":u32, "QE.STAT"=→"ENC.DIO_3.STAT":u8)  [unwired: 11 in]
    n227 = call "DIO_Encoder.vi"("DIO.1:0.OUT"=w484, "DIO.1:0.DIR"=w480, "QE.CNFG"="ENC.DIO_0.CNFG", "DIO.1/QE.B"=refnum<k21> "DIO/DIO1" ("DIO Refnum"), "SELECT"=w514, "DIO.0/QE.A"=refnum<k21> "DIO/DIO0" ("DIO Refnum")) -> ("DIO.1:0.IN"=w489:fxp<+,2,2>, "QE.CNTR"=→"ENC.DIO_0.CNTR":u32, "QE.STAT"=→"ENC.DIO_0.STAT":u8)  [unwired: 11 in]
    n228 = call "DIO_Encoder.vi"("DIO.1:0.OUT"=w483, "DIO.1:0.DIR"=w479, "QE.CNFG"="ENC.DIO_1.CNFG", "DIO.1/QE.B"=refnum<k21> "DIO/DIO3" ("DIO Refnum"), "SELECT"=w511, "DIO.0/QE.A"=refnum<k21> "DIO/DIO2" ("DIO Refnum")) -> ("DIO.1:0.IN"=w488:fxp<+,2,2>, "QE.CNTR"=→"ENC.DIO_1.CNTR":u32, "QE.STAT"=→"ENC.DIO_1.STAT":u8)  [unwired: 11 in]
    n229 = call "DIO_Encoder.vi"("DIO.1:0.OUT"=w482, "DIO.1:0.DIR"=w478, "QE.CNFG"="ENC.DIO_2.CNFG", "DIO.1/QE.B"=refnum<k21> "DIO/DIO5" ("DIO Refnum"), "SELECT"=w502, "DIO.0/QE.A"=refnum<k21> "DIO/DIO2" ("DIO Refnum")) -> ("DIO.1:0.IN"=w487:fxp<+,2,2>, "QE.CNTR"=→"ENC.DIO_2.CNTR":u32, "QE.STAT"=→"ENC.DIO_2.STAT":u8)  [unwired: 11 in]
    n230 = call "Join HDC Bank3 DIO.vi"("IN 7:6"=w472, "IN 5:4"=w487, "IN 3:2"=w488, "IN 1:0"=w489) -> ("OUT 7:0"=→"DIO.DIO_7:0.IN":u8)
    n231 = call "Split HDC Bank3 DIO.vi"("IN 7:0"="DIO.DIO_9:8.OUT") -> ("OUT 1:0"=w471:fxp<+,2,2>)  [unwired: 3 out]
    n232 = call "Split HDC Bank3 DIO.vi"("IN 7:0"="DIO.DIO_9:8.DIR") -> ("OUT 1:0"=w470:fxp<+,2,2>)  [unwired: 3 out]
    n233 = call "DIO_Encoder.vi"("DIO.1:0.OUT"=w471, "DIO.1:0.DIR"=w470, "QE.CNFG"="ENC.DIO_4.CNFG", "DIO.1/QE.B"=refnum<k21> "DIO/DIO9" ("DIO Refnum"), "SELECT"=w490, "DIO.0/QE.A"=refnum<k21> "DIO/DIO8" ("DIO Refnum")) -> ("DIO.1:0.IN"=w469:fxp<+,2,2>, "QE.CNTR"=→"ENC.DIO_4.CNTR":u32, "QE.STAT"=→"ENC.DIO_4.STAT":u8)  [unwired: 11 in]
    n234 = call "Join HDC Bank3 DIO.vi"("IN 1:0"=w469) -> ("OUT 7:0"=→"DIO.DIO_9:8.IN":u8)  [unwired: 3 in]
  }
  n235 = node-c288(w16) -> ()
  n236 = node-c288() -> (w21:T2)  [unwired: 1 in]
  n237 = timed-loop {
    timing: w21 -> [_]
    timing-out: [_] -> w20
    stop <- FALSE stop-if-true
    # "PWM1 were PWM8"
    # "First PWM1 were PWM0"
    # "PWM"
    n238 = call "PWM (Single Output).vi"("Clock Select"="PWM.PWM_0.CS", "Counter Control"="PWM.PWM_0.CNFG", "Output Compare Value"="PWM.PWM_0.CMP", "Max Counter Value"="PWM.PWM_0.MAX") -> ("Output"=w580:bool, "Counter Value"=→"PWM.PWM_0.CNTR":u16)  [unwired: 6 in]
    n239 = call "PWM (Single Output).vi"("Clock Select"="PWM.PWM_1.CS", "Counter Control"="PWM.PWM_1.CNFG", "Output Compare Value"="PWM.PWM_1.CMP", "Max Counter Value"="PWM.PWM_1.MAX") -> ("Output"=w574:bool, "Counter Value"=→"PWM.PWM_1.CNTR":u16)  [unwired: 6 in]
    n240 = call "PWM (Single Output).vi"("Clock Select"="PWM.PWM_2.CS", "Counter Control"="PWM.PWM_2.CNFG", "Output Compare Value"="PWM.PWM_2.CMP", "Max Counter Value"="PWM.PWM_2.MAX") -> ("Output"=w558:bool, "Counter Value"=→"PWM.PWM_2.CNTR":u16)  [unwired: 6 in]
    n241 = call "PWM (Single Output).vi"("Clock Select"="PWM.PWM_3.CS", "Counter Control"="PWM.PWM_3.CNFG", "Output Compare Value"="PWM.PWM_3.CMP", "Max Counter Value"="PWM.PWM_3.MAX") -> ("Output"=w557:bool, "Counter Value"=→"PWM.PWM_3.CNTR":u16)  [unwired: 6 in]
    n242 = call "PWM (Single Output).vi"("Clock Select"="PWM.PWM_4.CS", "Counter Control"="PWM.PWM_4.CNFG", "Output Compare Value"="PWM.PWM_4.CMP", "Max Counter Value"="PWM.PWM_4.MAX") -> ("Output"=w556:bool, "Counter Value"=→"PWM.PWM_4.CNTR":u16)  [unwired: 6 in]
    n243 = xnode "FPGA I/O Node"("PWM/PWM1"=w580, "PWM/PWM1"=w574, "PWM/PWM2"=w558, "PWM/PWM3"=w557, "PWM/PWM4"=w556) -> ()  [unwired: 5 in, 5 out]
    n244 = call "PWM (Single Output).vi"("Clock Select"="PWM.PWM_5.CS", "Counter Control"="PWM.PWM_5.CNFG", "Output Compare Value"="PWM.PWM_5.CMP", "Max Counter Value"="PWM.PWM_5.MAX") -> ("Output"=w531:bool, "Counter Value"=→"PWM.PWM_5.CNTR":u16)  [unwired: 6 in]
    n245 = call "PWM (Single Output).vi"("Clock Select"="PWM.PWM_6.CS", "Counter Control"="PWM.PWM_6.CNFG", "Output Compare Value"="PWM.PWM_6.CMP", "Max Counter Value"="PWM.PWM_6.MAX") -> ("Output"=w537:bool, "Counter Value"=→"PWM.PWM_6.CNTR":u16)  [unwired: 6 in]
    n246 = call "PWM (Single Output).vi"("Clock Select"="PWM.PWM_7.CS", "Counter Control"="PWM.PWM_7.CNFG", "Output Compare Value"="PWM.PWM_7.CMP", "Max Counter Value"="PWM.PWM_7.MAX") -> ("Output"=w553:bool, "Counter Value"=→"PWM.PWM_7.CNTR":u16)  [unwired: 6 in]
    n247 = call "PWM (Single Output).vi"("Clock Select"="PWM.PWM_8.CS", "Counter Control"="PWM.PWM_8.CNFG", "Output Compare Value"="PWM.PWM_8.CMP", "Max Counter Value"="PWM.PWM_8.MAX") -> ("Output"=w554:bool, "Counter Value"=→"PWM.PWM_8.CNTR":u16)  [unwired: 6 in]
    n248 = call "PWM (Single Output).vi"("Clock Select"="PWM.PWM_9.CS", "Counter Control"="PWM.PWM_9.CNFG", "Output Compare Value"="PWM.PWM_9.CMP", "Max Counter Value"="PWM.PWM_9.MAX") -> ("Output"=w555:bool, "Counter Value"=→"PWM.PWM_9.CNTR":u16)  [unwired: 6 in]
    n249 = xnode "FPGA I/O Node"("PWM/PWM5"=w531, "PWM/PWM6"=w537, "PWM/PWM7"=w553, "PWM/PWM1"=w554, "PWM/PWM9"=w555) -> ()  [unwired: 5 in, 5 out]
  }
  n250 = node-c288(w20) -> ()
  n251 = xnode "VI-Defined FIFO Configuration"() -> ("FIFO Out"=w6:refnum<k21>)
  n252 = node-c288() -> (w13:T2)  [unwired: 1 in]
  n253 = timed-loop {
    timing: w13 -> [_]
    timing-out: [_] -> w12
    tunnel: w6 -> [w590]
    stop <- FALSE stop-if-true
    # "SPI / CS DIO"
    # "SPI / SPI"
    # "SPI"
    n254 = xnode "FPGA I/O Node"() -> ("SPI MISO"=w607:bool)  [unwired: 1 in, 1 out]
    n255 = call "SPI Master.vi"("Count"="SPI.SPI.CNT", "Configuration"="SPI.SPI.CNFG", "Start?"="SPI.SPI.GO", "MISO"=w607, "Data Out"="SPI.SPI.DATO") -> ("Status"=w588:u8, "SCLK"=w601:bool, "MOSI"=w602:bool, "Data In"=→"SPI.SPI.DATI":u16)  [unwired: 3 in]
    "SPI.SPI.STAT" <- w588
    n256 = xnode "FPGA I/O Node"("SPI MOSI"=w602, "SPI CLK"=w601) -> ()  [unwired: 2 in, 2 out]
    n257 = call "SPI IRQ.vi"("SPI.A.IRQ.NO"="SPI.SPI.IRQ.NO", "SPI.STAT"=w588, "FIFO In"=w590) -> ()  [unwired: 9 in]
    n258 = call "Split HDC Bank1 DIO.vi"("IN 7:0"="DIO.SPI_CS3:0.OUT") -> ("OUT 3:0"=w597:fxp<+,4,4>)  [unwired: 2 out]
    n259 = call "Split HDC Bank1 DIO.vi"("IN 7:0"="DIO.SPI_CS3:0.DIR") -> ("OUT 3:0"=w596:fxp<+,4,4>)  [unwired: 2 out]
    n260 = call "DIO 4-bit.vi"("DIO0 Refnum"=refnum<k21> "SPI CS0", "DIO1 Refnum"=refnum<k21> "SPI CS1" ("DIO0 Refnum"), "DIO2 Refnum"=refnum<k21> "SPI CS2" ("DIO0 Refnum"), "DIR 3:0"=w596, "OUT 3:0"=w597, "DIO3 Refnum"=refnum<k21> "SPI CS3" ("DIO0 Refnum")) -> ("IN 3:0"=w595:fxp<+,4,4>)  [unwired: 5 in]
    n261 = call "Join HDC Bank1 DIO.vi"("IN 3:0"=w595) -> ("OUT 7:0"=→"DIO.SPI_CS3:0.IN":u8)  [unwired: 2 in]
  }
  n262 = while {
    stop <- FALSE stop-if-true
    # "Connector SPI SPI SCTL Interrupt Buffer"
    n263 = feedback #8(u8 0 ("Element")) -> (w614:u8)
    n264 = feedback #9(FALSE ("Timed Out?")) -> (w618:bool)
    n265 = case shown="False" w618 {
      tunnel: [w620 w622] -> w615
      tunnel: w614 -> [_ w622]
      frame False {
        n266 = xnode ("FIFO Method Node")("Timeout"=-1) -> ("Element"=w620:u8)  [unwired: 1 in, 2 out]
      }
      frame True {
      }
    }
    n267 = feedback-in #8(w615) -> ()
    n268 = xnode ("FIFO Method Node")("Element"=w615, "Timeout"=0) -> ("Timed Out?"=w616:bool)  [unwired: 1 in, 1 out]
    n269 = feedback-in #9(w616) -> ()
  }
  n270 = node-c288(w12) -> ()
  n271 = node-c288() -> (w15:T2)  [unwired: 1 in]
  n272 = timed-loop {
    timing: w15 -> [_]
    timing-out: [_] -> w14
    stop <- FALSE stop-if-true
    # "I2C"
    n273 = call "DIO_I2C.vi"("I2C.CNFG"="I2C.I2C.CNFG", "I2C.CNTL"="I2C.I2C.CNTL", "I2C.ADDR"="I2C.I2CADDR", "I2C.DATO"="I2C.I2C.DATO", "DIO.1/I2C.SDA"=refnum<k21> "I2C SDA" ("FPGA I/O In"), "I2C.CNTR"="I2C.I2C.CNTR", "DIO.0/I2C.SCL"=refnum<k21> "I2C SCL" ("FPGA I/O In"), "Execute?"="I2C.I2C.GO", "SELECT"=TRUE) -> ("I2C.DATI"=→"I2C.I2C.DATI":u8, "I2C.STAT"=→"I2C.I2C.STAT":u8)  [unwired: 8 in, 1 out]
  }
  n274 = node-c288(w14) -> ()
  n275 = node-c288() -> (w19:T2)  [unwired: 1 in]
  n276 = timed-loop {
    timing: w19 -> [_]
    timing-out: [_] -> w18
    stop <- FALSE stop-if-true
    # "Relay"
    n277 = Number To Boolean Array(number="DO.RELAY.OUT") -> (Boolean array=w645:bool[])
    n278 = Index Array(array=w645) -> (element #1=w644:bool, element #2=w643:bool, element #3=w642:bool, element #4=w641:bool, element #5=w640:bool, element #6=w639:bool, element #7=w638:bool, element #8=w637:bool)  [unwired: 8 in]
    n279 = xnode "FPGA I/O Node"("RelayFwd0"=w644, "RelayRev0"=w643, "RelayFwd1"=w642, "RelayRev1"=w641, "RelayFwd2"=w640, "RelayRev2"=w639, "RelayFwd3"=w638, "RelayRev3"=w637) -> ()  [unwired: 8 in, 8 out]
  }
  n280 = node-c288(w18) -> ()
  n281 = node-c288() -> (w11:T2)  [unwired: 1 in]
  n282 = timed-loop {
    timing: w11 -> [_]
    timing-out: [_] -> w10
    stop <- FALSE stop-if-true
    # "RSL"
    n283 = xnode "FPGA I/O Node"("RSL"="DO.RSL.OUT") -> ()  [unwired: 1 in, 1 out]
  }
  n284 = node-c288(w10) -> ()
